vi "Untitled 2.vi"() -> ()   [LabVIEW 2014]
panel:
  out "IQ":dbl
  out "R":dbl
  in  "y":dbl
  in  "x":dbl
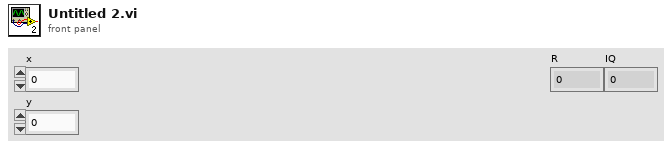
[diagram p1: front panel]
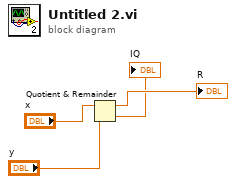
[diagram p0: block diagram]
diagram:
  n1 = Quotient & Remainder(x="x", y="y") -> (x-y*floor(x/y)=→"R":dbl, floor(x/y)=→"IQ":dbl)
